vi "Read Value.vi"(8 "error in (no error)":errorcluster caption="entrée d'erreur (pas d'erreur)", 11 "DAQmxTaskAICurrent_Emulate en entrée":refnum<class "DAQmxTaskAICurrent_Emulate.lvclass">) -> (0 "error out":errorcluster caption="sortie d'erreur", 1 "Data":bool, 2 "Data string":string, 3 "DAQmxTaskAICurrent_Emulate en sortie":refnum<class "DAQmxTaskAICurrent_Emulate.lvclass">)   [LabVIEW 2018, in "DAQmxTaskAICurrent_Emulate.lvclass"]
uses:
  DAQmxTaskAICurrent_Emulate.lvclass
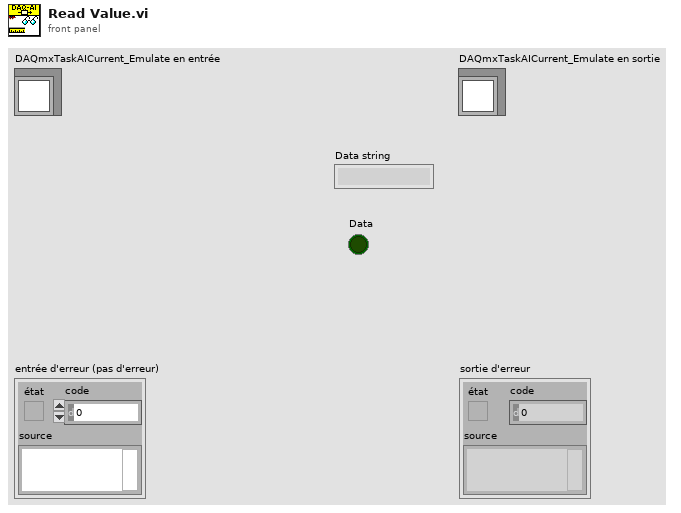
[diagram p1: front panel]
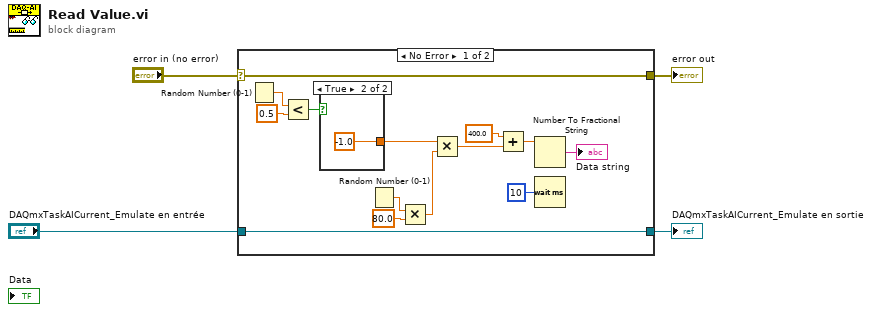
[diagram p0: block diagram]
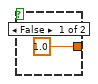
[diagram p2: hidden frame]
diagram:
  n1 = case shown="No Error" "error in (no error)" {
    selector: "error in (no error)" -> [w16 w22]
    tunnel: [w16 w22] -> w3
    tunnel: [w18 w21] -> w2
    tunnel: "DAQmxTaskAICurrent_Emulate en entrée" -> [w18 w21]
    frame No Error {
      n2 = Random Number (0-1)() -> (number: 0 to 1=w15:dbl)
      n3 = Less?(x=w15, y=0.5) -> (x < y?=w13:bool)
      n4 = case shown="True" w13 {
        tunnel: [1.0 -1.0] -> w12
        frame False {
        }
        frame True {
        }
      }
      n5 = Random Number (0-1)() -> (number: 0 to 1=w11:dbl)
      n6 = Multiply(x=w11, y=80.0) -> (x*y=w9:dbl)
      n7 = Multiply(x=w12, y=w9) -> (x*y=w7:dbl)
      n8 = Add(x=400.0, y=w7) -> (x+y=w6:dbl)
      n9 = Number To Fractional String(number=w6) -> (F-format string=→"Data string":string)  [unwired: 3 in]
      n10 = Wait (ms)(milliseconds to wait=u32 10) -> ()  [unwired: 1 out]
    }
    frame Error {
    }
  }
  "error out" <- w3
  "DAQmxTaskAICurrent_Emulate en sortie" <- w2
